vi "overPressureTest.vi"() -> ()   [LabVIEW 2021]
panel:
  out "Pressure":dbl[](graph)
  out "Voltage":dbl[](graph)
  out "Voltage Reading":dbl
  in  "Channel":u16
  out "Error Message":string
  out "Pressure Reading":dbl format="%.2f"
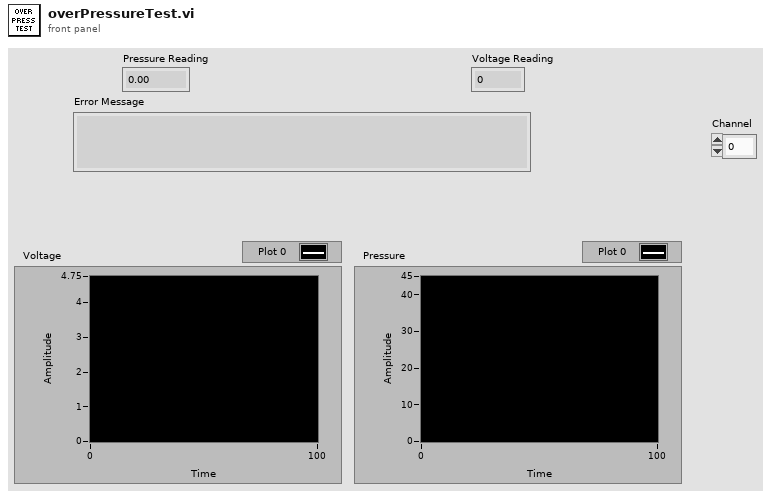
[diagram p1: front panel]
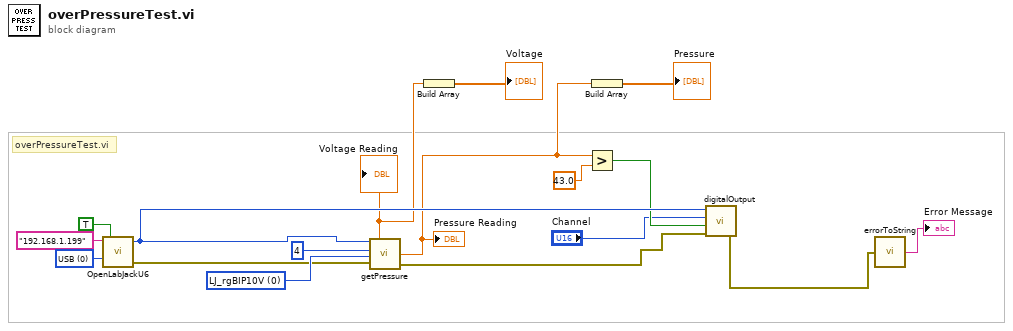
[diagram p0: block diagram]
diagram:
  w11 = u16 0 items=["LJ_rgBIP10V", "LJ_rgBIP5V", "LJ_rgUNI5V", "LJ_rgUNI2P5V", "LJ_rgUNI1P25V", "LJ_rgBIP1V", "LJ_rgUNIP625V", "LJ_rgBIPP1V", "LJ_rgBIPP01V"] ("AIN Range")
  w16 = u16 0 items=["USB", "Ethernet"] ("Connection Type")
  # "overPressureTest.vi"
  n1 = call "OpenLabJackU6.vi"("Select First Found"=TRUE, "Connection Type"=w16, "U6 Address"="192.168.1.199") -> ("error out"=w10:errorcluster, "Handle"=w9:i32)  [unwired: 1 in, 1 out]
  n2 = call "getPressure.vi"("error in"=w10, "AIN Range"=w11, "+Channel"=u16 4, "Handle In"=w9) -> ("error out"=w5:errorcluster, "Pressure Reading"=w4:dbl, "Voltage Reading"=w7:dbl)
  "Pressure Reading" <- w4
  "Voltage Reading" <- w7
  n3 = Build Array(w7) -> (→"Voltage":dbl[])
  n4 = Greater?(x=w4, y=43.0) -> (0:w3:bool)
  n5 = Build Array(w4) -> (→"Pressure":dbl[])
  n6 = call "digitalOutput.vi"("error in"=w5, "State"=w3, "Channel"="Channel", "Handle In"=w9) -> ("error out"=w1:errorcluster)  [unwired: 1 out]
  n7 = call "errorToString.vi"("error in"=w1) -> ("Error Message"=→"Error Message":string)
